vi "UV-VIS SetHSSpeedSD.vi"(4 "error in (no error)":errorcluster, 5 "index":i32, 6 "type":T1, 7 "Control in":refnum<class "CCD_camera.lvclass">) -> (0 "error out":errorcluster, 1 "DLL error code":u32, 3 "Control out":refnum<class "CCD_camera.lvclass">)   [LabVIEW 2015, in "CCD_camera.lvclass"]
doc: "This function will set the horizontal speed to one of the possible speeds of the system. It will be used for subsequent acquisitions.\n\n<B>Parameters:</B>\ntype - the horizontal read mode.\n Valid values: 0 - speed of data readout.\n 1 - speed of binning.\n 2 - speed of dumping pixels.\nindex - the horizontal speed to be used\n Valid values: 0 to <B>GetNumberHSSpeeds</B>-1\n\n<B>Error codes:</B>\nDRV_SUCCESS - Horizontal speed set.\nDRV_NOT_INITIALIZED - System not initialized.\nDRV_ACQUIRING - Acquisition in progress.\nDRV_P1INVALID - Mode is invalid.\nDRV_P2INVALID - Index is out off range."
uses:
  CCD_camera.lvclass
  atmcd32d.llb/HSSpeed_type typedef.ctl
  Detector.lvclass/Detector.ctl
  Detector.lvclass
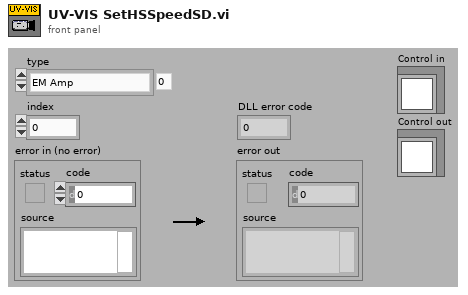
[diagram p1: front panel]
types:
  T1 = typedef "HSSpeed_type typedef.ctl" = enum16{"EM Amp", "Conventional Amp"}
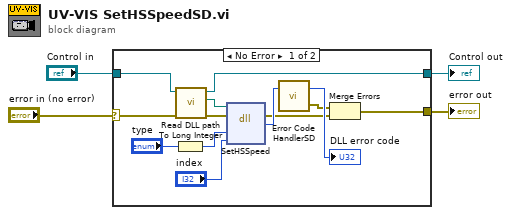
[diagram p0: block diagram]
diagram:
  n1 = case shown="No Error" "error in (no error)" {
    selector: "error in (no error)" -> [w11 w19]
    tunnel: [w6 w19] -> w3
    tunnel: [w5 w18] -> w2
    tunnel: "Control in" -> [w12 w18]
    frame No Error {
      n2 = To Long Integer(number="type") -> (32bit integer=w14:i32)
      n3 = call "Read DLL path.vi"("error in (no error)"=w11, "Detector in"=w12) -> ("error out"=w10:errorcluster, "DLL path"=w9:path, "Detector out"=w5:refnum<class "CCD_camera.lvclass">)  [unwired: 7 in]
      n4 = dll-call lib="S:/TRANCON/DLL/Atmcd32d.dll" fn="SetHSSpeed"(path in=w9, error in=w10, "type"=w14, "index"="index") -> (error out=w8:errorcluster, "return type"=w17:u32)  [unwired: 3 in, 1 out]
      n5 = call "Error Code HandlerSD.vi"("DLL error code"=w17) -> ("error out"=w7:errorcluster, "dup DLL error code"=→"DLL error code":u32)  [unwired: 1 in]
      n6 = Merge Errors(w7, w8) -> (w6:errorcluster)
    }
    frame Error {
    }
  }
  "error out" <- w3
  "Control out" <- w2
